vi "Update Panels in Device List.vi"(5 "Old List":u16[](array[numeric]), 7 "New List":u16[](array[numeric]), 8 "Error In":errorcluster, 11 "Device List State":T1) -> (0 "Error Out":errorcluster, 3 "Device List State out":T1)   [LabVIEW 2015]
uses:
  Device List State.ctl
  Device/Device.lvclass
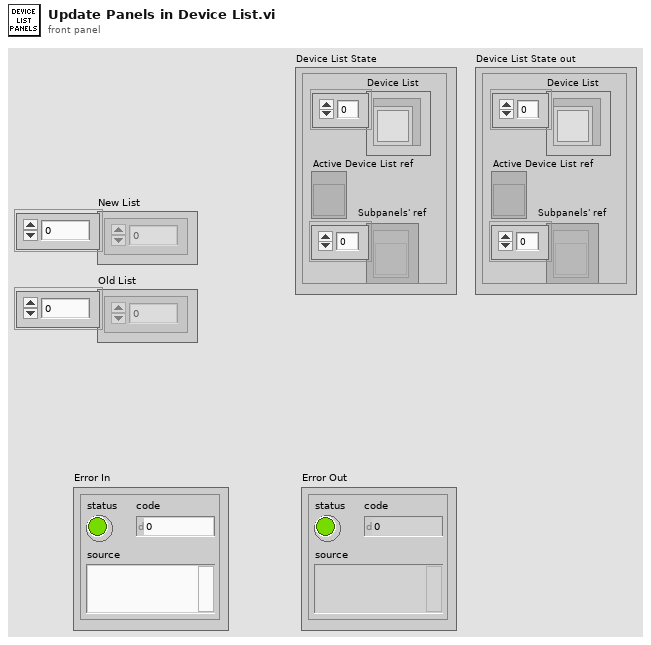
[diagram p1: front panel]
types:
  T1 = typedef "Device List State.ctl" = cluster{"Device List":refnum<class "Device.lvclass">[], "Active Device List ref":refnum<vi>, "Subpanels' ref":refnum<vi>[]}
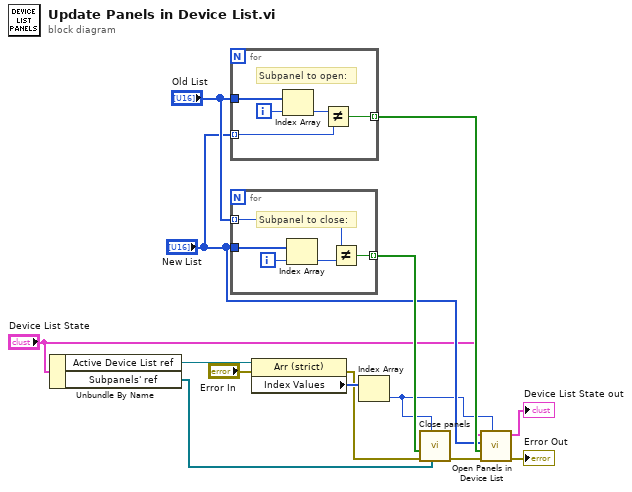
[diagram p0: block diagram]
diagram:
  n1 = Unbundle By Name("Device List State") -> ("Active Device List ref"=w1:refnum<vi>, "Subpanels' ref"=w3:refnum<vi>[])
  n2 = for {
    tunnel: "New List" -> [w15] mode=indexing
    tunnel: "Old List" -> [w18]
    tunnel: [w17] -> w8 mode=indexing
    i -> [w19]
    # "Subpanel to open:"
    n3 = Index Array(array=w18, index=w19) -> (element=w16:u16)
    n4 = Not Equal?(x=w16, y=w15) -> (x != y?=w17:bool)
  }
  n5 = for {
    tunnel: "Old List" -> [w22] mode=indexing
    tunnel: "New List" -> [w23]
    tunnel: [w20] -> w12 mode=indexing
    i -> [w24]
    # "Subpanel to close:"
    n6 = Index Array(array=w23, index=w24) -> (element=w21:u16)
    n7 = Not Equal?(x=w22, y=w21) -> (x != y?=w20:bool)
  }
  n8 = property on="Property Node" class="Arr (strict)"(reference=w1, error in="Error In") -> (error out=w11:errorcluster, "Index Values"=w13:u32[])  [unwired: 1 out]
  n9 = Index Array(array=w13) -> (element=w6:u32)  [unwired: 1 in]
  n10 = call "Close panels.vi"("Subpanels' ref"=w3, "Index Value"=w6, "error in (no error)"=w11, "Subpanels to close"=w12) -> ("error out"=w9:errorcluster)  [unwired: 7 in]
  n11 = call "Open Panels in Device List.vi"("Index Value"=w6, "error in (no error)"=w9, "Subpanels to open"=w8, "Active List"="New List", "Device List State"="Device List State") -> ("error out"=→"Error Out":errorcluster, "Device List State out"=→"Device List State out":T1)  [unwired: 5 in]
